vi "ttm_run2.vi"(0 "protocolName":string, 1 "channelInt":i32, 2 "rampRateAE":dbl, 3 "rampRateSilent":dbl, 4 "timeWindow":dbl, 5 "cycleLength":dbl, 6 "holdTime":dbl, 7 "expId":string, 9 "rampRate":dbl, 10 "load":dbl, 11 "rampAmplitude":dbl) -> (20 "protocolNameOut":string, 21 "channelIntOut":i32)   [LabVIEW 2009]
panel:
  out "loggingOnOut":bool
  out "expIdOut":string
  out "startLoggingOut":bool
  in  "?":enum32{"AEcontrol", "Cyclic", "Ramp", "Creep"}(tab)
  out "timeWindowOut":dbl
  out "rampRateSilentOut":dbl
  out "rampRateAEout":dbl
  out "startAeControlOut":bool=TRUE
  out "aeControlRunningOut":bool=TRUE
  out "rampAmplitudeOut":dbl
  out "rampRateOut":dbl
  out "startSetRampOut":bool
  out "startRampOut":bool
  out "startCreepOut":bool
  out "creepRunningOut":bool
  out "creepLoadOut":dbl
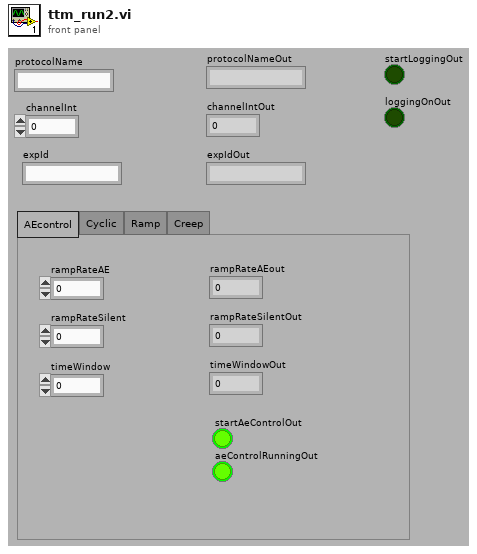
[diagram p1: front panel]
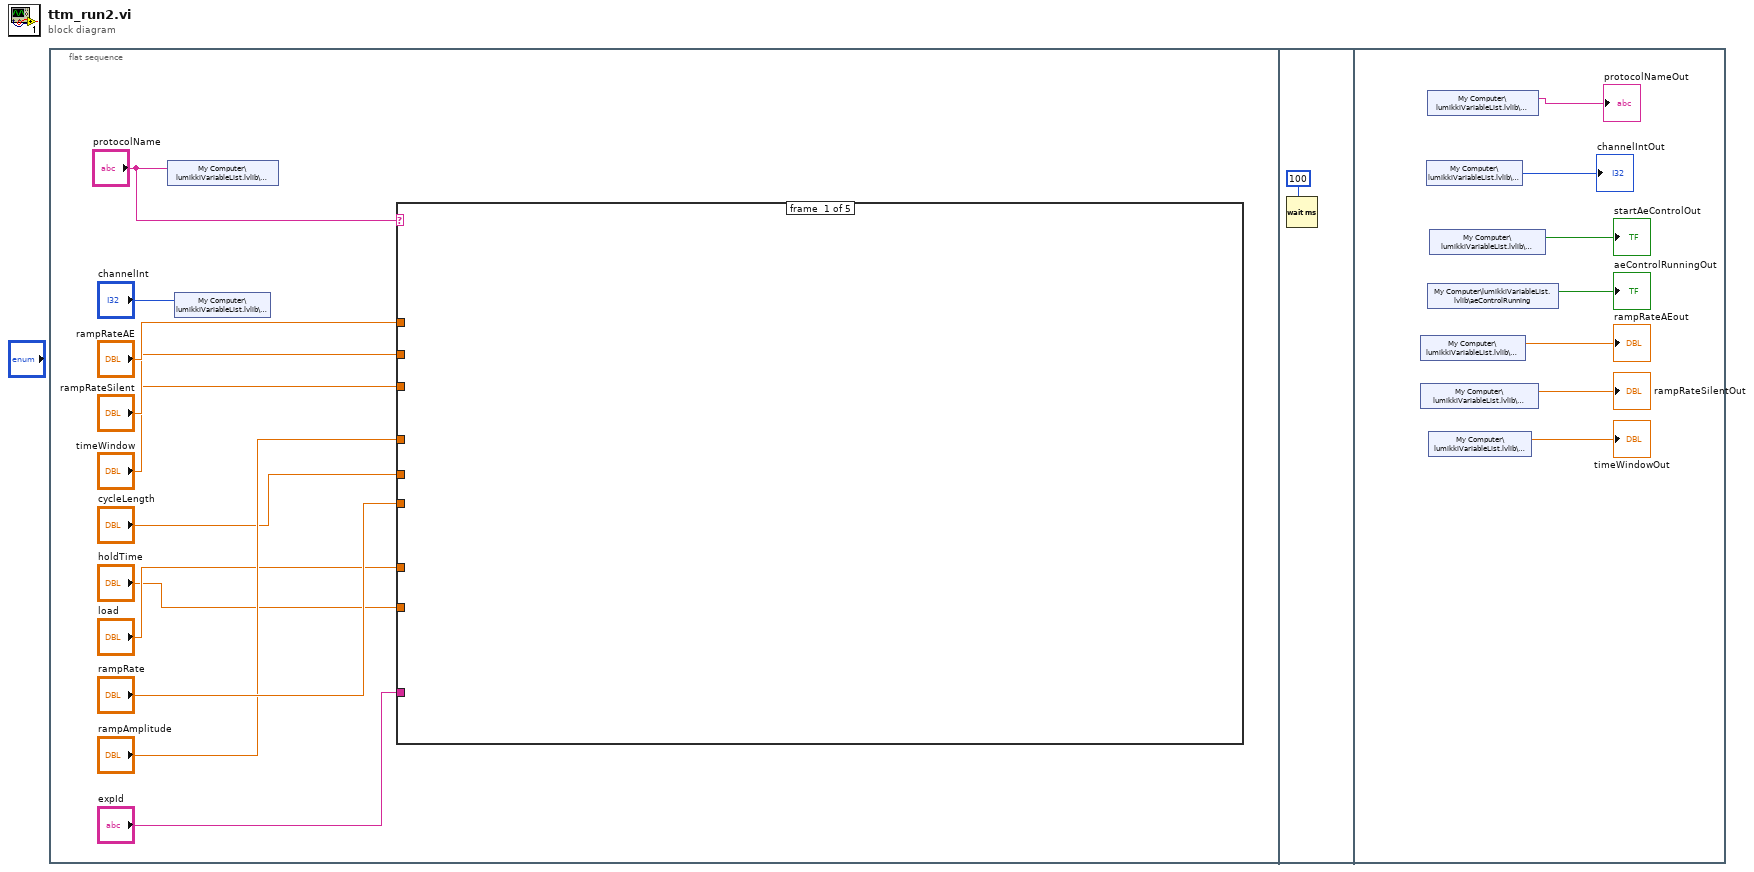
[diagram p0: block diagram]
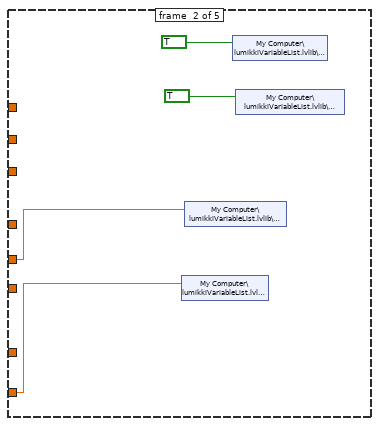
[diagram p2: hidden frame]
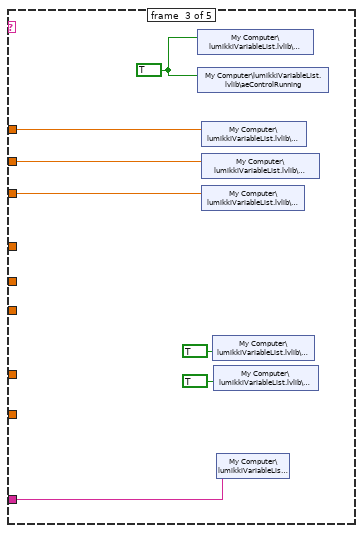
[diagram p3: hidden frame]
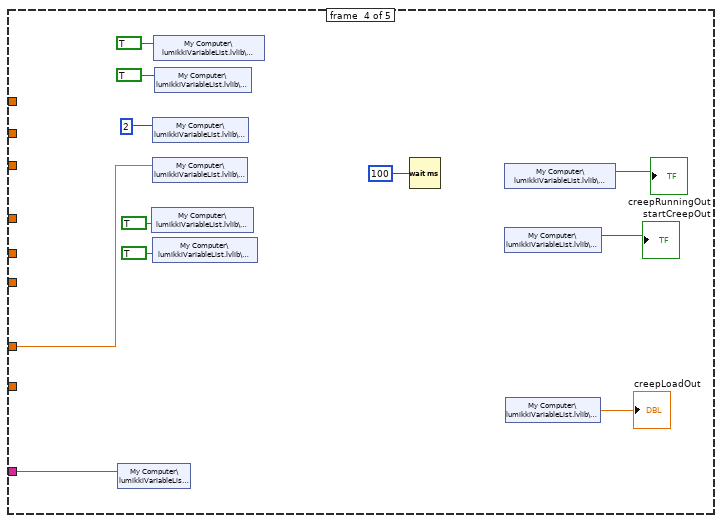
[diagram p4: hidden frame]
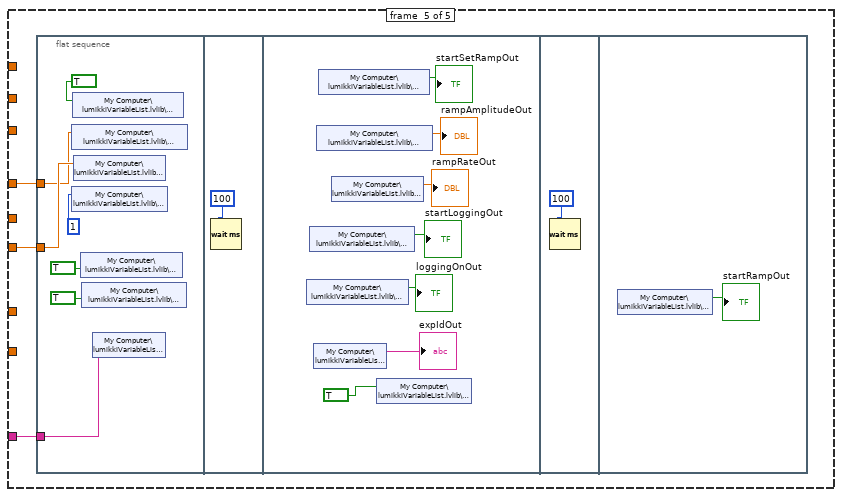
[diagram p5: hidden frame]
diagram:
  n1 = flat-sequence {
    frame #0 {
      n2 = shared-variable "My Computer\\lumikkiVariableList.lvlib\\protocolName"("protocolName") -> ()  [unwired: 1 in, 1 out]
      n3 = shared-variable "My Computer\\lumikkiVariableList.lvlib\\channelInt"("channelInt") -> ()  [unwired: 1 in, 1 out]
      n4 = case shown="\"tensile\"" "protocolName" {
        tunnel: "rampRateAE" -> [_ _ w21 _ _]
        tunnel: "rampRateSilent" -> [_ _ w20 _ _]
        tunnel: "timeWindow" -> [_ _ w19 _ _]
        tunnel: "rampRate" -> [_ _ _ _ w36]
        tunnel: "rampAmplitude" -> [_ _ _ _ w35]
        tunnel: "expId" -> [_ _ w16 w33 w34]
        tunnel: "load" -> [_ _ _ w23 _]
        tunnel: "cycleLength" -> [_ w13 _ _ _]
        tunnel: "holdTime" -> [_ w12 _ _ _]
        frame #0 {
        }
        frame #1 {
          n5 = shared-variable "My Computer\\lumikkiVariableList.lvlib\\holdTime"(w12) -> ()  [unwired: 1 in, 1 out]
          n6 = shared-variable "My Computer\\lumikkiVariableList.lvlib\\cycleLength"(w13) -> ()  [unwired: 1 in, 1 out]
          n7 = shared-variable "My Computer\\lumikkiVariableList.lvlib\\startCyclic"(TRUE) -> ()  [unwired: 1 in, 1 out]
          n8 = shared-variable "My Computer\\lumikkiVariableList.lvlib\\cyclicRunning"(TRUE) -> ()  [unwired: 1 in, 1 out]
        }
        frame #2 {
          w22 = TRUE
          n9 = shared-variable "My Computer\\lumikkiVariableList.lvlib\\startAeControl"(w22) -> ()  [unwired: 1 in, 1 out]
          n10 = shared-variable "My Computer\\lumikkiVariableList.lvlib\\aeControlRunning"(w22) -> ()  [unwired: 1 in, 1 out]
          n11 = shared-variable "My Computer\\lumikkiVariableList.lvlib\\rampRateAE"(w21) -> ()  [unwired: 1 in, 1 out]
          n12 = shared-variable "My Computer\\lumikkiVariableList.lvlib\\rampRateSilent"(w20) -> ()  [unwired: 1 in, 1 out]
          n13 = shared-variable "My Computer\\lumikkiVariableList.lvlib\\timeWindow"(w19) -> ()  [unwired: 1 in, 1 out]
          n14 = shared-variable "My Computer\\lumikkiVariableList.lvlib\\loggingIsOn"(TRUE ("Busy")) -> ()  [unwired: 1 in, 1 out]
          n15 = shared-variable "My Computer\\lumikkiVariableList.lvlib\\startLogging"(TRUE ("Busy")) -> ()  [unwired: 1 in, 1 out]
          n16 = shared-variable "My Computer\\lumikkiVariableList.lvlib\\expId"(w16) -> ()  [unwired: 1 in, 1 out]
        }
        frame #3 {
          n17 = shared-variable "My Computer\\lumikkiVariableList.lvlib\\expId"(w33) -> ()  [unwired: 1 in, 1 out]
          n18 = shared-variable "My Computer\\lumikkiVariableList.lvlib\\loggingIsOn"(TRUE ("Busy")) -> ()  [unwired: 1 in, 1 out]
          n19 = shared-variable "My Computer\\lumikkiVariableList.lvlib\\channelInt"(2) -> ()  [unwired: 1 in, 1 out]
          n20 = shared-variable "My Computer\\lumikkiVariableList.lvlib\\creepLoad"(w23) -> ()  [unwired: 1 in, 1 out]
          n21 = shared-variable "My Computer\\lumikkiVariableList.lvlib\\startLogging"(TRUE ("Busy")) -> ()  [unwired: 1 in, 1 out]
          n22 = shared-variable "My Computer\\lumikkiVariableList.lvlib\\creepRunning"(TRUE ("Busy")) -> ()  [unwired: 1 in, 1 out]
          n23 = shared-variable "My Computer\\lumikkiVariableList.lvlib\\startCreep"(TRUE ("Busy")) -> ()  [unwired: 1 in, 1 out]
          n24 = Wait (ms)(milliseconds to wait=u32 100) -> ()  [unwired: 1 out]
          n25 = shared-variable "My Computer\\lumikkiVariableList.lvlib\\creepRunning"() -> (→"creepRunningOut":bool)  [unwired: 1 in, 1 out]
          n26 = shared-variable "My Computer\\lumikkiVariableList.lvlib\\startCreep"() -> (→"startCreepOut":bool)  [unwired: 1 in, 1 out]
          n27 = shared-variable "My Computer\\lumikkiVariableList.lvlib\\creepLoad"() -> (→"creepLoadOut":dbl)  [unwired: 1 in, 1 out]
        }
        frame #4 {
          n28 = flat-sequence {
            tunnel: w36 -> [w41]
            tunnel: w35 -> [w40]
            tunnel: w34 -> [w37]
            frame #0 {
              n29 = shared-variable "My Computer\\lumikkiVariableList.lvlib\\rampAmplitude"(w40) -> ()  [unwired: 1 in, 1 out]
              n30 = shared-variable "My Computer\\lumikkiVariableList.lvlib\\channelInt"(1 ("channelInt")) -> ()  [unwired: 1 in, 1 out]
              n31 = shared-variable "My Computer\\lumikkiVariableList.lvlib\\startSetRamp"(TRUE ("Busy")) -> ()  [unwired: 1 in, 1 out]
              n32 = shared-variable "My Computer\\lumikkiVariableList.lvlib\\rampRate"(w41) -> ()  [unwired: 1 in, 1 out]
              n33 = shared-variable "My Computer\\lumikkiVariableList.lvlib\\loggingIsOn"(TRUE ("Busy")) -> ()  [unwired: 1 in, 1 out]
              n34 = shared-variable "My Computer\\lumikkiVariableList.lvlib\\startLogging"(TRUE ("Busy")) -> ()  [unwired: 1 in, 1 out]
              n35 = shared-variable "My Computer\\lumikkiVariableList.lvlib\\expId"(w37) -> ()  [unwired: 1 in, 1 out]
            }
            frame #1 {
              n36 = Wait (ms)(milliseconds to wait=u32 100) -> ()  [unwired: 1 out]
            }
            frame #2 {
              n37 = shared-variable "My Computer\\lumikkiVariableList.lvlib\\loggingIsOn"() -> (→"loggingOnOut":bool)  [unwired: 1 in, 1 out]
              n38 = shared-variable "My Computer\\lumikkiVariableList.lvlib\\startLogging"() -> (→"startLoggingOut":bool)  [unwired: 1 in, 1 out]
              n39 = shared-variable "My Computer\\lumikkiVariableList.lvlib\\expId"() -> (→"expIdOut":string)  [unwired: 1 in, 1 out]
              n40 = shared-variable "My Computer\\lumikkiVariableList.lvlib\\rampAmplitude"() -> (→"rampAmplitudeOut":dbl)  [unwired: 1 in, 1 out]
              n41 = shared-variable "My Computer\\lumikkiVariableList.lvlib\\startSetRamp"() -> (→"startSetRampOut":bool)  [unwired: 1 in, 1 out]
              n42 = shared-variable "My Computer\\lumikkiVariableList.lvlib\\rampRate"() -> (→"rampRateOut":dbl)  [unwired: 1 in, 1 out]
              n43 = shared-variable "My Computer\\lumikkiVariableList.lvlib\\startRamp"(TRUE ("Busy")) -> ()  [unwired: 1 in, 1 out]
            }
            frame #3 {
              n44 = Wait (ms)(milliseconds to wait=u32 100) -> ()  [unwired: 1 out]
            }
            frame #4 {
              n45 = shared-variable "My Computer\\lumikkiVariableList.lvlib\\startRamp"() -> (→"startRampOut":bool)  [unwired: 1 in, 1 out]
            }
          }
        }
      }
    }
    frame #1 {
      n46 = Wait (ms)(milliseconds to wait=u32 100) -> ()  [unwired: 1 out]
    }
    frame #2 {
      n47 = shared-variable "My Computer\\lumikkiVariableList.lvlib\\rampRateAE"() -> (→"rampRateAEout":dbl)  [unwired: 1 in, 1 out]
      n48 = shared-variable "My Computer\\lumikkiVariableList.lvlib\\rampRateSilent"() -> (→"rampRateSilentOut":dbl)  [unwired: 1 in, 1 out]
      n49 = shared-variable "My Computer\\lumikkiVariableList.lvlib\\channelInt"() -> (→"channelIntOut":i32)  [unwired: 1 in, 1 out]
      n50 = shared-variable "My Computer\\lumikkiVariableList.lvlib\\protocolName"() -> (→"protocolNameOut":string)  [unwired: 1 in, 1 out]
      n51 = shared-variable "My Computer\\lumikkiVariableList.lvlib\\aeControlRunning"() -> (→"aeControlRunningOut":bool)  [unwired: 1 in, 1 out]
      n52 = shared-variable "My Computer\\lumikkiVariableList.lvlib\\timeWindow"() -> (→"timeWindowOut":dbl)  [unwired: 1 in, 1 out]
      n53 = shared-variable "My Computer\\lumikkiVariableList.lvlib\\startAeControl"() -> (→"startAeControlOut":bool)  [unwired: 1 in, 1 out]
    }
  }
